vi "Example JSON Difference.vi"() -> ()   [LabVIEW 2015]
uses:
  JSONtext.lvlib
panel:
  out "First File":path
  out "Second File":path
  out "<JSON> 2":string caption="<JSON>Changes (Second from First)"
  out "<JSON>":string caption="<JSON>Changes (First from Second)"
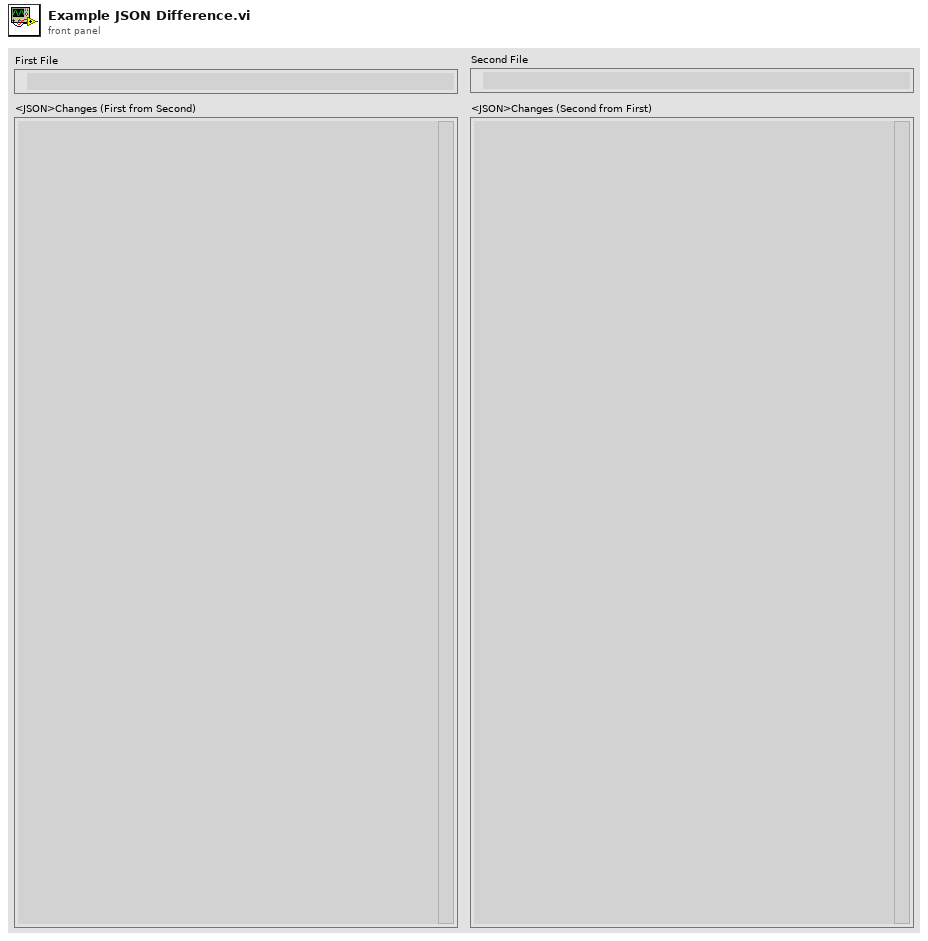
[diagram p1: front panel]
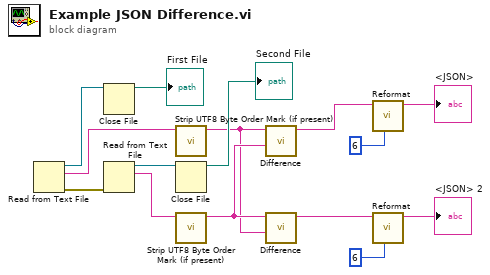
[diagram p0: block diagram]
diagram:
  n1 = Read from Text File() -> (refnum out=w7:refnum<file>, text=w4:string, error out=w15:errorcluster)  [unwired: 4 in, 1 out]
  n2 = Close File(refnum=w7) -> (path=→"First File":path)  [unwired: 1 in, 1 out]
  n3 = Read from Text File(error in=w15) -> (refnum out=w10:refnum<file>, text=w6:string)  [unwired: 3 in, 2 out]
  n4 = call "Strip UTF8 Byte Order Mark (if present).vi"("Text in"=w4) -> ("Possible Byte Order Mark Stripped"=w3:string)  [unwired: 10 in]
  n5 = Close File(refnum=w10) -> (path=→"Second File":path)  [unwired: 1 in, 1 out]
  n6 = call "Strip UTF8 Byte Order Mark (if present).vi"("Text in"=w6) -> ("Possible Byte Order Mark Stripped"=w5:string)  [unwired: 10 in]
  n7 = call "Difference.vi"("Compare to this JSON Object"=w5, "JSON Object"=w3) -> ("<JSON>"=w14:string)  [unwired: 7 in, 1 out]
  n8 = call "Difference.vi"("Compare to this JSON Object"=w3, "JSON Object"=w5) -> ("<JSON>"=w1:string)  [unwired: 7 in, 1 out]
  n9 = call "Reformat.vi"("Pretty Print Levels"=6, "Input String"=w14) -> ("<JSON>First JSON Value"=→"<JSON>":string)  [unwired: 6 in, 3 out]
  n10 = call "Reformat.vi"("Pretty Print Levels"=6, "Input String"=w1) -> ("<JSON>First JSON Value"=→"<JSON> 2":string)  [unwired: 6 in, 3 out]
